vi "Configure Trigger Model Delta Block.vi"(0 "VISA resource name":refnum<visa-resource-name>, 1 "Block Number (1)":i32=1 min=1 format="%#.6g", 2 "Target Difference (0)":dbl format="%#.6g", 3 "Branch Path (1)":i32=1 min=1 format="%#.6g", 4 "Measure Block (1)":i32=1 min=1 format="%#.6g", 5 "error in (no error)":errorcluster) -> (14 "VISA resource name out":refnum<visa-resource-name>, 19 "error out":errorcluster)   [LabVIEW 2018, in "Keithley 2450.lvlib"]
doc: "This VI defines a trigger model block that goes to a specified block if the difference of two measurements meets preset criteria."
uses:
  <instrlib>/Keithley 2450/Keithley 2450.lvlib
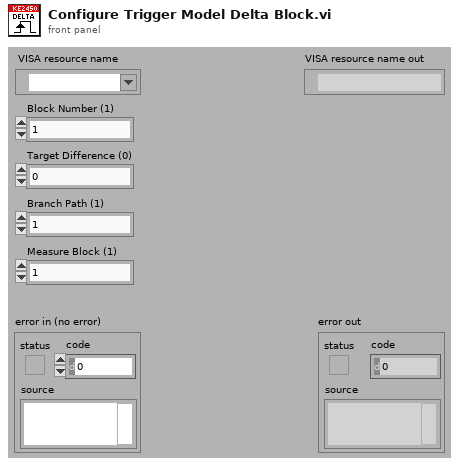
[diagram p1: front panel]
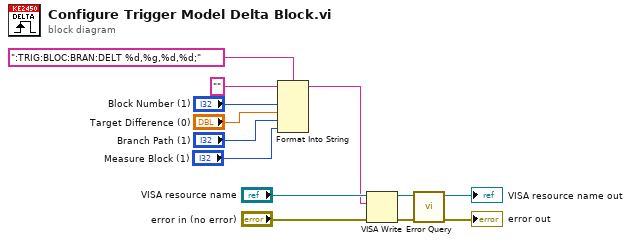
[diagram p0: block diagram]
diagram:
  n1 = Format Into String(format string=":TRIG:BLOC:BRAN:DELT %d,%g,%d,%d;", initial string="", "Block Number (1)", "Target Difference (0)", "Branch Path (1)", "Measure Block (1)") -> (resulting string=w4:string)  [unwired: 1 in, 1 out]
  n2 = VISA Write(VISA resource name="VISA resource name", write buffer=w4, error in (no error)="error in (no error)") -> (VISA resource name out=w9:refnum<visa-resource-name>, error out=w8:errorcluster)  [unwired: 1 out]
  n3 = call <instrlib>:"Error Query.vi"("error in (no error)"=w8, "VISA resource name"=w9) -> ("error out"=→"error out":errorcluster, "VISA resource name out"=→"VISA resource name out":refnum<visa-resource-name>)  [unwired: 8 out]
